vi "FPGA_convert_U8-to-fix-bool-array.vi"(11 "U8":u8) -> (1 "bool array":bool[](array[boolean]))   [LabVIEW 2013]
panel:
  # "Converts a U8 to a bool array in fixed size array"
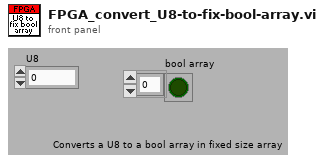
[diagram p1: front panel]
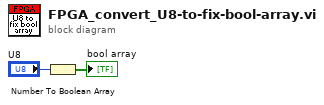
[diagram p0: block diagram]
diagram:
  n1 = Number To Boolean Array(number="U8") -> (Boolean array=→"bool array":bool[])
